vi "bnomoveY.vi"(8 "error in (no error)":errorcluster, 11 "Y":dbl) -> (0 "error out":errorcluster)   [LabVIEW 2019]
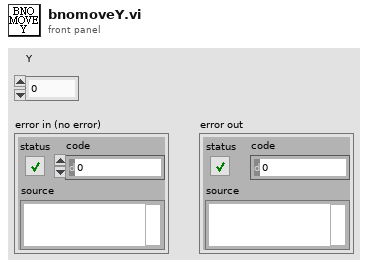
[diagram p1: front panel]
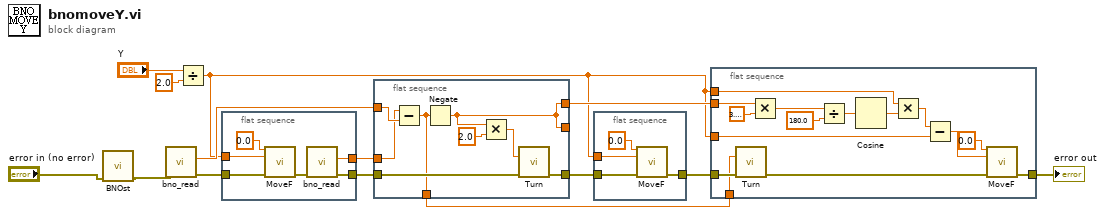
[diagram p0: block diagram]
diagram:
  n1 = call "BNOst.vi"("error in (no error)"="error in (no error)") -> ("error out"=w2:errorcluster)  [unwired: 10 in]
  n2 = call "bno_read.vi"("error in (no error)"=w2) -> ("error out"=w7:errorcluster, "x/y"=w8:dbl)  [unwired: 8 in]
  n3 = Divide(x="Y", y=2.0) -> (x/y=w4:dbl)
  n4 = flat-sequence {
    tunnel: w7 -> [w20]
    tunnel: w4 -> [w19]
    tunnel: [w16] -> w13
    tunnel: [w15] -> w14
    frame #0 {
      n5 = call "MoveF.vi"("X"=0.0, "Y"=w19, "error in (no error)"=w20) -> ("error out"=w17:errorcluster)  [unwired: 12 in]
      n6 = call "bno_read.vi"("error in (no error)"=w17) -> ("error out"=w16:errorcluster, "x/y"=w15:dbl)  [unwired: 8 in]
    }
  }
  n7 = flat-sequence {
    tunnel: w8 -> [w28]
    tunnel: [w22] -> w11
    tunnel: [w27] -> w5
    tunnel: w13 -> [w26]
    tunnel: w14 -> [w25]
    tunnel: [w22] -> _
    tunnel: [w21] -> w1
    frame #0 {
      n8 = Subtract(x=w25, y=w28) -> (x-y=w21:dbl)
      n9 = Negate(x=w21) -> (-x=w22:dbl)
      n10 = Multiply(x=w22, y=2.0) -> (x*y=w23:dbl)
      n11 = call "Turn.vi"("¨¤«×"=w23, "error in (no error)"=w26) -> ("error out"=w27:errorcluster)  [unwired: 13 in]
    }
  }
  n12 = flat-sequence {
    tunnel: [w32] -> w6
    tunnel: w5 -> [w31]
    tunnel: w4 -> [w29]
    frame #0 {
      n13 = call "MoveF.vi"("X"=0.0, "Y"=w29, "error in (no error)"=w31) -> ("error out"=w32:errorcluster)  [unwired: 12 in]
    }
  }
  n14 = flat-sequence {
    tunnel: w4 -> [w47]
    tunnel: w11 -> [w45]
    tunnel: [w38] -> w12
    tunnel: w4 -> [w34]
    tunnel: w6 -> [w36]
    tunnel: w1 -> [w33]
    frame #0 {
      n15 = call "Turn.vi"("¨¤«×"=w33, "error in (no error)"=w36) -> ("error out"=w37:errorcluster)  [unwired: 13 in]
      n16 = Multiply(x=w45, y=3.141592653589793) -> (x*y=w41:dbl)
      n17 = Divide(x=w41, y=180.0) -> (x/y=w39:dbl)
      n18 = Cosine(x=w39) -> (cos(x)=w46:dbl)
      n19 = Multiply(x=w47, y=w46) -> (x*y=w35:dbl)
      n20 = Subtract(x=w35, y=w34) -> (x-y=w40:dbl)
      n21 = call "MoveF.vi"("X"=0.0, "Y"=w40, "error in (no error)"=w37) -> ("error out"=w38:errorcluster)  [unwired: 12 in]
    }
  }
  "error out" <- w12
